vi "Odbior danych z PC .vi"(8 "error in (no error)":errorcluster, 11 "connection ID":refnum<k16>) -> (0 "error out":errorcluster, 3 "connection ID out":refnum<k16>, 5 "Output Data":T1)   [LabVIEW 2015]
uses:
  PC/QMH Fundamentals - Message Cluster.ctl
  <vilib>/RioEmbeddedCAN/RioEmbeddedCAN.llb/CANFrameControl.ctl
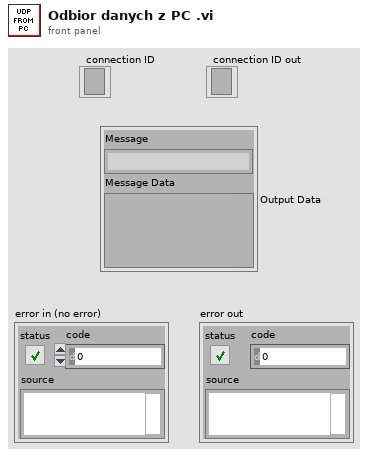
[diagram p1: front panel]
types:
  T1 = typedef "QMH Fundamentals - Message Cluster.ctl" = cluster{"Message":string, "Message Data":variant}
  T2 = typedef "CANFrameControl.ctl" = cluster{"identifier":u32, "extended?":bool, "type":u8, "payload":u8[]}
  T3 = cluster{"Data":cluster{"date/time string":string, "array of cans":T2[]}, "bool":bool}
  T4 = cluster{"date/time string":string, "array of cans":T2[]}
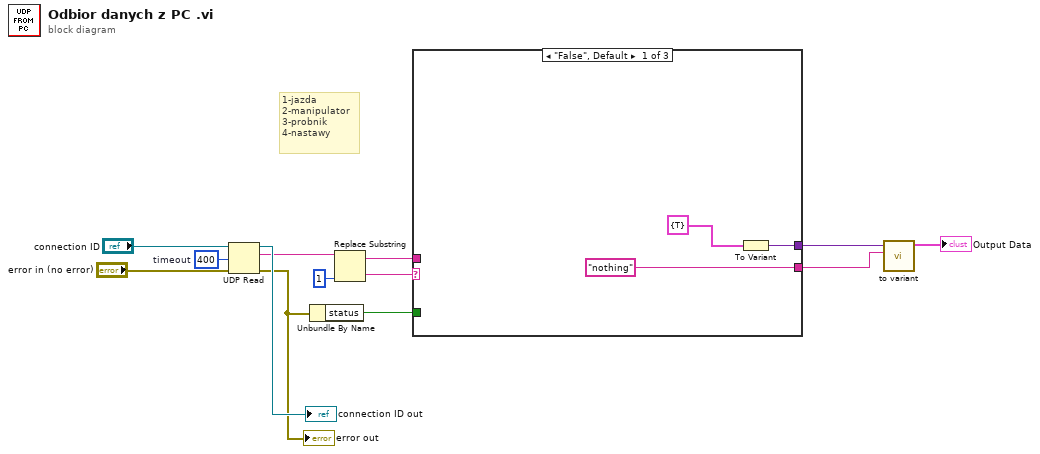
[diagram p0: block diagram]
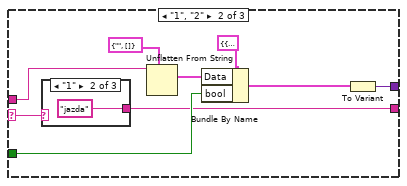
[diagram p2: hidden frame]
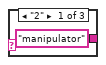
[diagram p3: hidden frame]
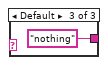
[diagram p4: hidden frame]
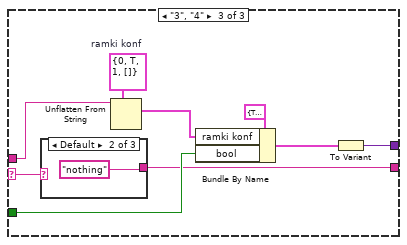
[diagram p5: hidden frame]
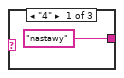
[diagram p6: hidden frame]
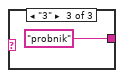
[diagram p7: hidden frame]
diagram:
  w11 = 400  # timeout
  # "1-jazda\n2-manipulator\n3-probnik\n4-nastawy"
  n1 = UDP Read(connection ID="connection ID", timeout ms (25000)=w11, 8:"error in (no error)") -> (data out=w8:string, error out=w5:errorcluster, 3:→"connection ID out":refnum<k16>)  [unwired: 1 in, 2 out]
  "error out" <- w5
  n2 = Unbundle By Name(w5) -> ("status"=w4:bool)
  n3 = Replace Substring(2:1 ("length (len. of substring)"), 5:w8) -> (0:w7:string, 1:w6:string)  [unwired: 2 in]
  n4 = case shown="\"False\", Default" w7 {
    selector: w7 -> [_ w21 w35]
    tunnel: w6 -> [_ w24 w36]
    tunnel: w4 -> [_ w20 w32]
    tunnel: ["nothing" w19 w31] -> w2
    tunnel: [w15 w18 w29] -> w1
    frame "False", Default {
      n5 = To Variant(anything=cluster{bool} {TRUE}) -> (Variant=w15:variant)
    }
    frame "1", "2" {
      n6 = case shown="\"1\"" w21 {
        tunnel: ["manipulator" "jazda" "nothing"] -> w19
        frame "2" {
        }
        frame "1" {
        }
        frame Default {
        }
      }
      n7 = Unflatten From String(type=T4 {"date/time string"="", "array of cans"=[]} ("output cluster"), binary string=w24) -> (value=w23:T4)  [unwired: 3 in, 2 out]
      n8 = Bundle By Name(cluster=T3 {"Data"={"date/time string"="", "array of cans"=[]}, "bool"=TRUE} ("jazda"), "Data"=w23, "bool"=w20) -> (w17:T3)
      n9 = To Variant(anything=w17) -> (Variant=w18:variant)
    }
    frame "3", "4" {
      w37 = T2 {"identifier"=0, "extended?"=TRUE, "type"=1, "payload"=[]}  # ramki konf
      n10 = case shown="Default" w35 {
        tunnel: ["nastawy" "nothing" "probnik"] -> w31
        frame "4" {
        }
        frame Default {
        }
        frame "3" {
        }
      }
      n11 = Unflatten From String(type=w37, binary string=w36) -> (value=w33:T2)  [unwired: 3 in, 2 out]
      n12 = Bundle By Name(cluster=cluster{"bool":bool, "ramki konf":T2} {"bool"=TRUE, "ramki konf"={"identifier"=0, "extended?"=TRUE, "type"=1, "payload"=[]}} ("jazda"), "ramki konf"=w33, "bool"=w32) -> (w30:cluster{"bool":bool, "ramki konf":T2})
      n13 = To Variant(anything=w30) -> (Variant=w29:variant)
    }
  }
  n14 = call "to variant.vi"("Message"=w2, "Variant"=w1) -> ("Message Cluster"=→"Output Data":T1)  [unwired: 9 in]
